vi "Sign Test (median).vi"(6 "alternative hypothesis":i32(ring) items=["median(pop) != median"=0, "median(pop) > median"=1, "median(pop) < median"=-1], 9 "significance level":dbl=0.05, 10 "median":dbl, 11 "sample set":dbl[](array[numeric])) -> (0 "error":i32, 2 "p value":dbl=0.05 format="%.6g", 3 "reject null hypothesis":bool)   [LabVIEW 2018, in "NI_Gmath.lvlib"]
doc: "Tests hypotheses about the <B>median</B> of continuous distributions. You must manually select the polymorphic instance to use."
uses:
  NI_Gmath.lvlib
panel:
  # "Sign Test"
  # "null hypothesis\nmedian(pop) = median"
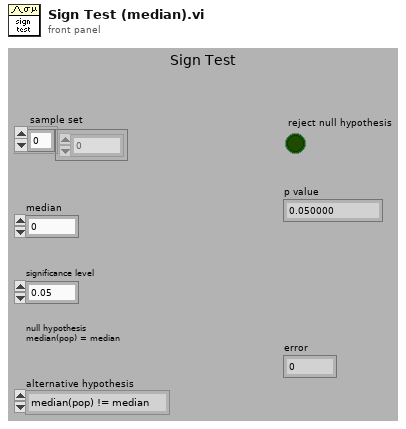
[diagram p1: front panel]
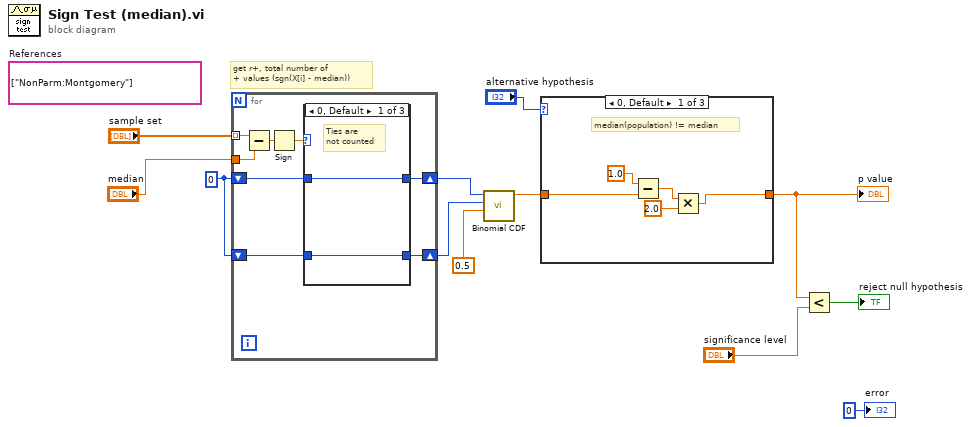
[diagram p0: block diagram]
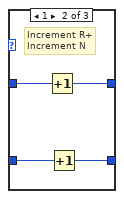
[diagram p2: hidden frame]
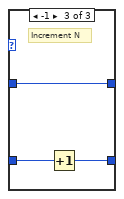
[diagram p3: hidden frame]
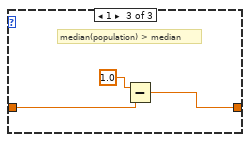
[diagram p5: hidden frame]
diagram:
  (unwired) string[] ["NonParm:Montgomery"]  # References
  w3 = 0
  # "get r+, total number of\n+ values (sgn(X[i] - median))"
  n1 = for {
    shift-right: [w15] -> w1
    shift-left: w3 -> [w16]
    shift-right: [w17] -> w2
    shift-left: w3 -> [w18]
    tunnel: "sample set" -> [w14] mode=indexing
    tunnel: "median" -> [w13]
    n2 = Subtract(x=w14, y=w13) -> (x-y=w20:dbl)
    n3 = Sign(1:w20) -> (0:w19:dbl)
    n4 = case shown="0, Default" w19 {
      tunnel: w18 -> [w22 w24 w29]
      tunnel: [w22 w23 w28] -> w17
      tunnel: w16 -> [w21 w26 w27]
      tunnel: [w21 w25 w27] -> w15
      frame 0, Default {
        # "Ties are\nnot counted"
      }
      frame 1 {
        # "Increment R+\nIncrement N"
        n5 = Increment(x=w26) -> (x+1=w25:i32)
        n6 = Increment(x=w24) -> (x+1=w23:i32)
      }
      frame -1 {
        # "Increment N"
        n7 = Increment(x=w29) -> (x+1=w28:i32)
      }
    }
  }
  n8 = call "Binomial CDF.vi"("p"=0.5 ("a"), "n"=w2, "x"=w1) -> ("cdf(x)"=w7:dbl)  [unwired: 7 in, 1 out]
  n9 = case shown="0, Default" "alternative hypothesis" {
    tunnel: [w31 w35 w37] -> w11
    tunnel: w7 -> [w30 w35 w36]
    frame 0, Default {
      # "median(population) != median"
      n10 = Subtract(x=1.0, y=w30) -> (x-y=w32:dbl)
      n11 = Multiply(x=w32, y=2.0) -> (x*y=w31:dbl)
    }
    frame -1 {
      # "median(population) < median"
    }
    frame 1 {
      # "median(population) > median"
      n12 = Subtract(x=1.0, y=w36) -> (x-y=w37:dbl)
    }
  }
  "p value" <- w11
  n13 = Less?(x=w11, y="significance level") -> (x < y?=→"reject null hypothesis":bool)
  "error" <- 0 ("error")
